vi "wczytanie ini test.vi"() -> ()   [LabVIEW 2014]
uses:
  Kontrolki/KartaDAQ/A_B konfig params.ctl
  <vilib>/Utility/config.llb/NI_LVConfig.lvlib
panel:
  out "HW params":T1={"wsp A"=[[924.40878695, 280.05044565000003, 29.1408959, 3.069102995, 0.31092278139], [914.0777918499999, 281.867210667, 26.882632206700002, 3.0550163421, 0.310968736845], [951.1456429000001, 285.110341112, 27.1990911426, 3.0696112628, 0.31581308595], [914.3476122000001, 281.34234172, 29.109892152, 3.068518068, 0.3126783], [1000.257513479, 304.977147369, 29.713910529099998, 3.0892035357, 0.31184511849999996], [993.0576890607, 303.5092078312, 29.442198783999, 3.0648262983400003, 0.31009064088000005], [1002.5166520152, 305.28578467799997, 29.440497145920002, 3.07102698336, 0.30933858648], [992.737407739, 302.6919371861, 29.47518592865, 3.0793274388799996, 0.31143866215]], "wsp B"=[[924.40878695, 280.05044565000003, 29.1408959, 3.069102995, 0.31092278139], [914.0777918499999, 281.867210667, 26.882632206700002, 3.0550163421, 0.310968736845], [951.1456429000001, 285.110341112, 27.1990911426, 3.0696112628, 0.31581308595], [914.3476122000001, 281.34234172, 29.109892152, 3.068518068, 0.3126783], [1000.257513479, 304.977147369, 29.713910529099998, 3.0892035357, 0.31184511849999996], [993.0576890607, 303.5092078312, 29.442198783999, 3.0648262983400003, 0.31009064088000005], [1002.5166520152, 305.28578467799997, 29.440497145920002, 3.07102698336, 0.30933858648], [992.737407739, 302.6919371861, 29.47518592865, 3.0793274388799996, 0.31143866215]]}
  in  "odwroc?":bool
  out "mb":dbl
  out "ma":dbl
  out "kb":dbl[](array[numeric])
  out "ka":dbl[](array[numeric])
  out "karty b":dbl[][](array[numeric])
  out "karty a":dbl[][](array[numeric])
  out "Wzmocnienia":dbl[][](array[numeric])
  in  "Path ini":path=path "C:/Users/user/Documents/Rejestrator/Konfiguracja/dev_27150498.jnj"
  out "mainboiard a":dbl[](array[numeric])
  out "Karty":dbl[][](array[numeric])
  out "mainboiard b":dbl[](array[numeric])
  out "error out":errorcluster
  in  "error in (no error)":errorcluster
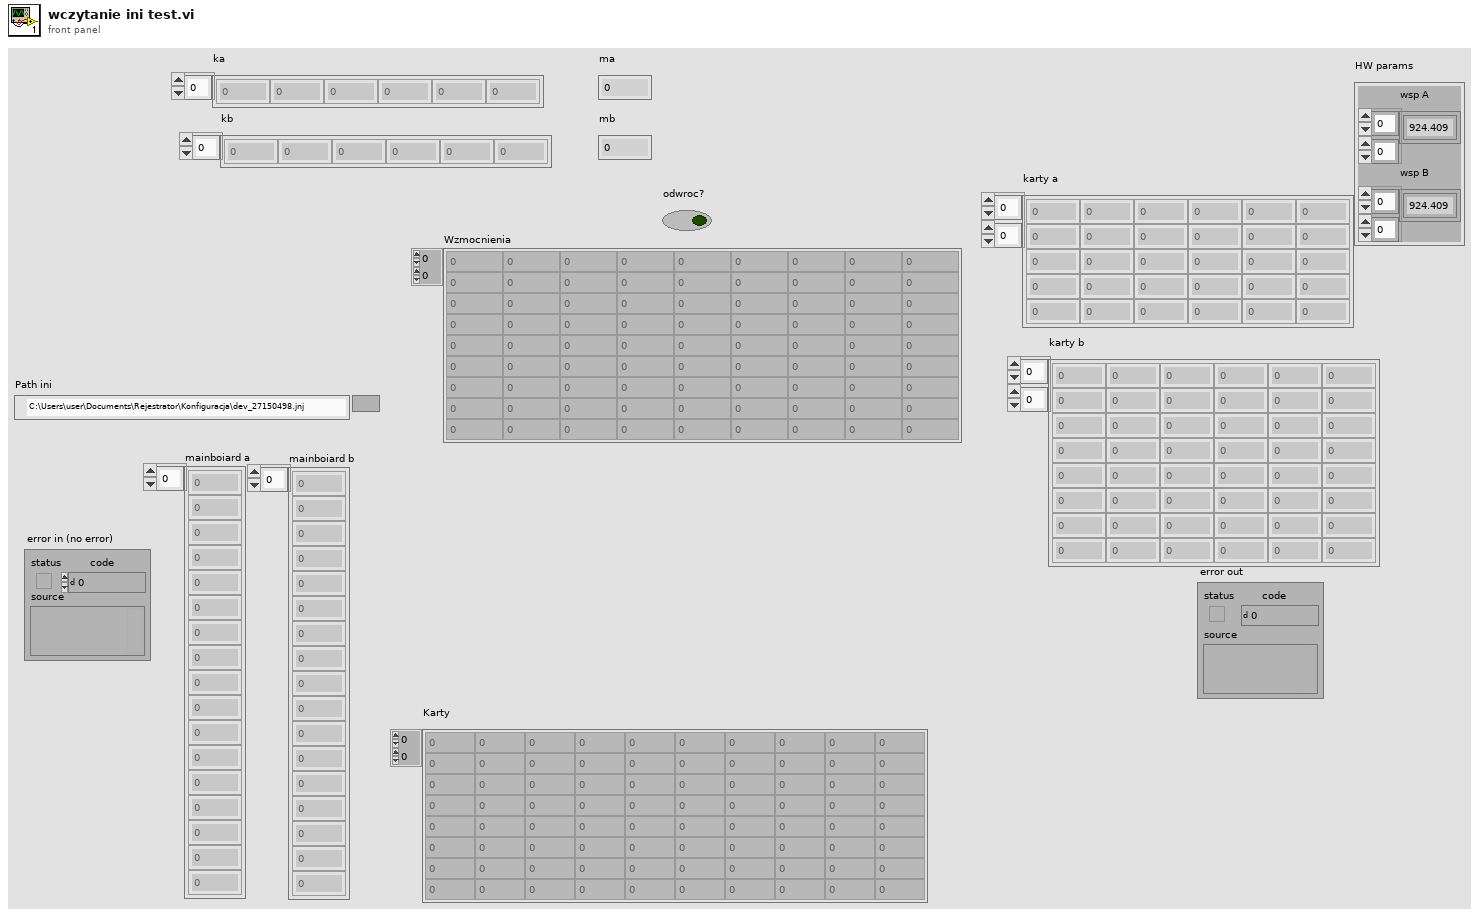
[diagram p1: front panel]
types:
  T1 = typedef "A_B konfig params.ctl" = cluster{"wsp A":dbl[][], "wsp B":dbl[][]}
  T2 = typedef "NI_LVConfig.lvlib/Config Data RefNum.ctl" = refnum<k1>
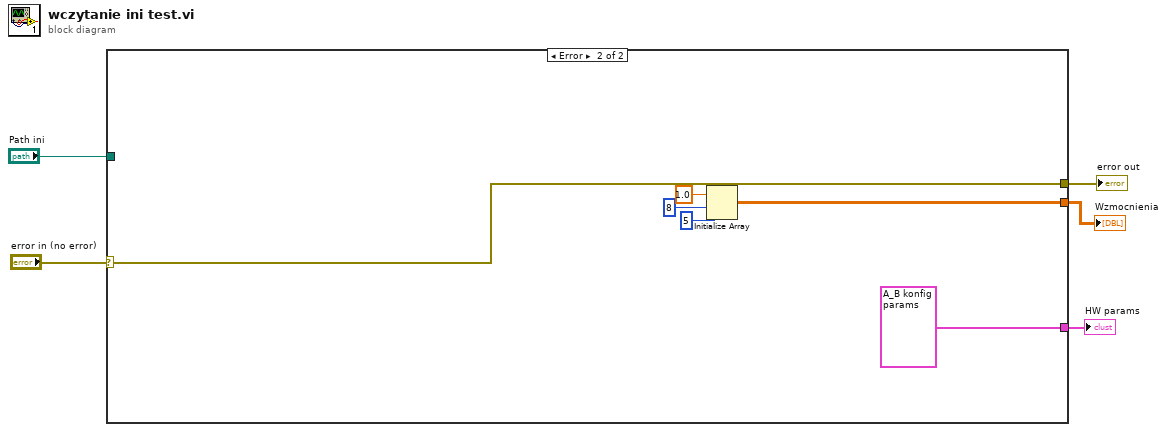
[diagram p0: block diagram]
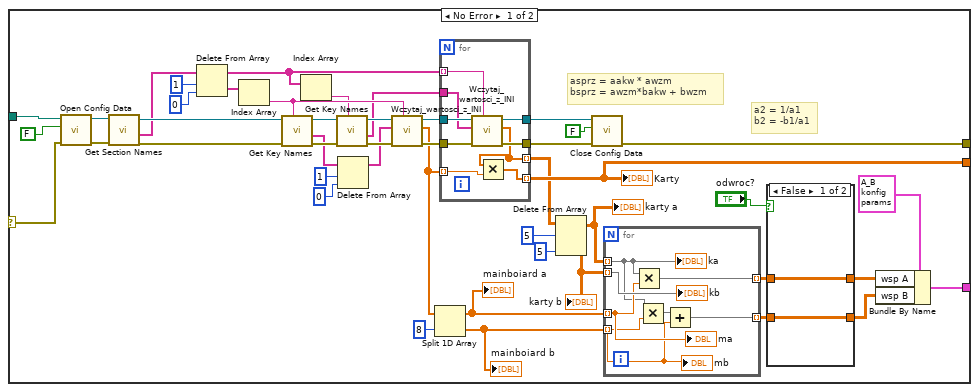
[diagram p2: hidden frame]
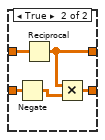
[diagram p3: hidden frame]
diagram:
  n1 = case shown="Error" "error in (no error)" {
    selector: "error in (no error)" -> [w50 w80]
    tunnel: [w44 w80] -> w4
    tunnel: "Path ini" -> [w51 _]
    tunnel: [w21 w76] -> w2
    tunnel: [w6 T1 {"wsp A"=[[924.40878695, 280.05044565000003, 29.1408959, 3.069102995, 0.31092278139], [914.0777918499999, 281.867210667, 26.882632206700002, 3.0550163421, 0.310968736845], [951.1456429000001, 285.110341112, 27.1990911426, 3.0696112628, 0.31581308595], [914.3476122000001, 281.34234172, 29.109892152, 3.068518068, 0.3126783], [1000.257513479, 304.977147369, 29.713910529099998, 3.0892035357, 0.31184511849999996], [993.0576890607, 303.5092078312, 29.442198783999, 3.0648262983400003, 0.31009064088000005], [1002.5166520152, 305.28578467799997, 29.440497145920002, 3.07102698336, 0.30933858648], [992.737407739, 302.6919371861, 29.47518592865, 3.0793274388799996, 0.31143866215]], "wsp B"=[[924.40878695, 280.05044565000003, 29.1408959, 3.069102995, 0.31092278139], [914.0777918499999, 281.867210667, 26.882632206700002, 3.0550163421, 0.310968736845], [951.1456429000001, 285.110341112, 27.1990911426, 3.0696112628, 0.31581308595], [914.3476122000001, 281.34234172, 29.109892152, 3.068518068, 0.3126783], [1000.257513479, 304.977147369, 29.713910529099998, 3.0892035357, 0.31184511849999996], [993.0576890607, 303.5092078312, 29.442198783999, 3.0648262983400003, 0.31009064088000005], [1002.5166520152, 305.28578467799997, 29.440497145920002, 3.07102698336, 0.30933858648], [992.737407739, 302.6919371861, 29.47518592865, 3.0793274388799996, 0.31143866215]]}] -> w1
    frame No Error {
      # "a2 = 1/a1\nb2 = -b1/a1"
      # "asprz = aakw * awzm\nbsprz = awzm*bakw + bwzm"
      n2 = call <vilib>:"Open Config Data.vi"("error in (no error)"=w50, "create file if necessary (T)"=FALSE, "configuration file path"=w51) -> ("error out"=w47:errorcluster, "refnum"=w48:T2)  [unwired: 6 in, 1 out]
      n3 = call <vilib>:"Get Section Names.vi"("error in (no error)"=w47, "refnum"=w48) -> ("error out"=w45:errorcluster, "section names"=w40:string[], "refnum out"=w46:T2)  [unwired: 7 in]
      n4 = Delete From Array ("section names")(array=w40, length=1, index=0) -> (deleted portion=w39:string[], array with subset deleted=w28:string[])
      n5 = Index Array(array=w39) -> (element=w34:string)  [unwired: 1 in]
      n6 = call <vilib>:"Get Key Names.vi"("section"=w34, "error in (no error)"=w45, "refnum"=w46) -> ("error out"=w33:errorcluster, "key names"=w25:string[], "refnum out"=w32:T2)  [unwired: 5 in, 1 out]
      n7 = Index Array(array=w28) -> (element=w29:string)  [unwired: 1 in]
      n8 = call <vilib>:"Get Key Names.vi"("section"=w29, "error in (no error)"=w33, "refnum"=w32) -> ("error out"=w31:errorcluster, "key names"=w23:string[], "refnum out"=w30:T2)  [unwired: 5 in, 1 out]
      n9 = Delete From Array(array=w25, length=1, index=0) -> (array with subset deleted=w24:string[])  [unwired: 1 out]
      n10 = call "Wczytaj_wartosci_z_INI.vi"("Section"=w34, "error in (no error)"=w31, "key names"=w24, "refnum"=w30) -> ("error out"=w38:errorcluster, "Array"=w14:dbl[], "refnum out"=w37:T2)  [unwired: 5 in]
      n11 = Split 1D Array(array=w14, index=8) -> (first subarray=w16:dbl[], second subarray=w15:dbl[])
      "mainboiard a" <- w16
      "mainboiard b" <- w15
      n12 = for {
        tunnel: w38 -> [w74]
        tunnel: w37 -> [w73]
        tunnel: [w71] -> w36
        tunnel: w28 -> [w70] mode=indexing
        tunnel: w23 -> [w69]
        tunnel: [w72] -> w35
        tunnel: [w68] -> w21 mode=indexing
        tunnel: w14 -> [w67] mode=indexing
        tunnel: [w66] -> w13 mode=indexing
        n13 = call "Wczytaj_wartosci_z_INI.vi"("Section"=w70, "error in (no error)"=w74, "key names"=w69, "refnum"=w73) -> ("error out"=w72:errorcluster, "Array"=w66:dbl[], "refnum out"=w71:T2)  [unwired: 5 in]
        n14 = Multiply(x=w66, y=w67) -> (x*y=w68:dbl[])
      }
      "Karty" <- w21
      n15 = Delete From Array(array=w13, length=5, index (col)=5 ("disabled index (col)")) -> (deleted portion=w17:dbl[][], array with subset deleted=w18:dbl[][])  [unwired: 1 in]
      "karty a" <- w18
      "karty b" <- w17
      n16 = call <vilib>:"Close Config Data.vi"("error in (no error)"=w35, "write file if changed (T)"=FALSE, "refnum"=w36) -> ("error out"=w44:errorcluster)  [unwired: 7 in, 1 out]
      n17 = for {
        tunnel: w18 -> [w62] mode=indexing
        tunnel: w17 -> [w65] mode=indexing
        tunnel: w16 -> [w64] mode=indexing
        tunnel: w15 -> [w60] mode=indexing
        tunnel: [w63] -> w12 mode=indexing
        tunnel: [w59] -> w11 mode=indexing
        n18 = Multiply(x=w62, y=w64) -> (x*y=w63:dbl[])
        n19 = Multiply(x=w62, y=w60) -> (x*y=w61:dbl[])
        n20 = Add(x=w61, y=w60) -> (x+y=w59:dbl[])
        "ka" <- w62
        "kb" <- w65
        "ma" <- w64
        "mb" <- w60
      }
      n21 = case shown="False" "odwroc?" {
        tunnel: w12 -> [w53 w58]
        tunnel: [w53 w54] -> w8
        tunnel: w11 -> [w52 w57]
        tunnel: [w52 w56] -> w7
        frame False {
        }
        frame True {
          n22 = Negate(x=w57) -> (-x=w55:dbl[][])
          n23 = Reciprocal(x=w58) -> (1/x=w54:dbl[][])
          n24 = Multiply(x=w54, y=w55) -> (x*y=w56:dbl[][])
        }
      }
      n25 = Bundle By Name(cluster=T1 {"wsp A"=[[924.40878695, 280.05044565000003, 29.1408959, 3.069102995, 0.31092278139], [914.0777918499999, 281.867210667, 26.882632206700002, 3.0550163421, 0.310968736845], [951.1456429000001, 285.110341112, 27.1990911426, 3.0696112628, 0.31581308595], [914.3476122000001, 281.34234172, 29.109892152, 3.068518068, 0.3126783], [1000.257513479, 304.977147369, 29.713910529099998, 3.0892035357, 0.31184511849999996], [993.0576890607, 303.5092078312, 29.442198783999, 3.0648262983400003, 0.31009064088000005], [1002.5166520152, 305.28578467799997, 29.440497145920002, 3.07102698336, 0.30933858648], [992.737407739, 302.6919371861, 29.47518592865, 3.0793274388799996, 0.31143866215]], "wsp B"=[[924.40878695, 280.05044565000003, 29.1408959, 3.069102995, 0.31092278139], [914.0777918499999, 281.867210667, 26.882632206700002, 3.0550163421, 0.310968736845], [951.1456429000001, 285.110341112, 27.1990911426, 3.0696112628, 0.31581308595], [914.3476122000001, 281.34234172, 29.109892152, 3.068518068, 0.3126783], [1000.257513479, 304.977147369, 29.713910529099998, 3.0892035357, 0.31184511849999996], [993.0576890607, 303.5092078312, 29.442198783999, 3.0648262983400003, 0.31009064088000005], [1002.5166520152, 305.28578467799997, 29.440497145920002, 3.07102698336, 0.30933858648], [992.737407739, 302.6919371861, 29.47518592865, 3.0793274388799996, 0.31143866215]]}, "wsp A"=w8, "wsp B"=w7) -> (w6:T1)
    }
    frame Error {
      n26 = Initialize Array(1.0 ("element"), 8 ("dimension size"), 5 ("dimension size")) -> (w76:dbl[][])
    }
  }
  "error out" <- w4
  "Wzmocnienia" <- w2
  "HW params" <- w1
